vi "UHR-Fleezers Control (host) - 12.1_Jonathan.vi"() -> ()   [LabVIEW 2012] (continued)
        n2038 = xnode "Read/Write Control"("FPGA VI Reference In"=w3388, "error in"=w3383, "FB Reset Set 1"=w3386, "FB Reset Set 2"=w3385) -> ("error out"=w3384:errorcluster)  [unwired: 1 out]
      }
      event "PID Gains": Value Change {
        n2039 = event-data() -> ()  [unwired: 7 out]
        n2040 = Unbundle By Name("PID Gains") -> ("Set 1"=w3392:T15, "Set 2"=w3391:T15)
        n2041 = xnode "Read/Write Control"("FPGA VI Reference In"=w3393, "error in"=w3389, "FB Gains Set 1"=w3392, "FB Gains Set 2"=w3391) -> ("error out"=w3390:errorcluster)  [unwired: 1 out]
      }
      event "AI2 to Setpoint", "Setpoints (V)": Value Change {
        n2042 = event-data() -> ()  [unwired: 7 out]
        n2043 = xnode "Read/Write Control"("FPGA VI Reference In"=w3399, "error in"=w3395) -> ("FPGA VI Reference Out"=w3398:T20, "error out"=w3397:errorcluster, "AI2 Y Sum Set 1"=w3406:i16, "AI2 Y Sum Set 2"=w3405:i16)
        n2044 = Cluster To Array(cluster="AI2 to Setpoint") -> (array=w3409:bool[])
        n2045 = local read "AI2 (V)"() -> (w3407:cluster{"Set 1":dbl, "Set 2":dbl})
        n2046 = Or Array Elements(Boolean array=w3409) -> (logical OR=w3410:bool)
        n2047 = Bundle By Name(cluster=w3407, "Set 1"=w3406, "Set 2"=w3405) -> (w3404:cluster{"Set 1":dbl, "Set 2":dbl})
        n2048 = Divide(x=w3404, y=3276.7) -> (x/y=w3403:cluster{"Set 1":dbl, "Set 2":dbl})
        "AI2 (V)" <- w3403
        n2049 = case shown="True" w3410 {
          tunnel: [w3413 w3430] -> w3402
          tunnel: "AI2 to Setpoint" -> [_ w3426]
          tunnel: "Setpoints (V)" -> [w3414 w3429]
          tunnel: w3403 -> [_ w3423]
          frame False {
            n2050 = Multiply(x=3276.7, y=w3414) -> (x*y=w3415:cluster{"Set 1":dbl, "Set 2":dbl})
            n2051 = To Word Integer(number=w3415) -> (16bit integer=w3413:cluster{"Set 1":i16, "Set 2":i16})
          }
          frame True {
            n2052 = Unbundle By Name(w3423) -> ("Set 1"=w3422:dbl, "Set 2"=w3421:dbl)
            n2053 = Unbundle By Name(w3429) -> ("Set 1"=w3428:dbl, "Set 2"=w3427:dbl)
            n2054 = Unbundle By Name(w3426) -> ("Set 1"=w3425:bool, "Set 2"=w3424:bool)
            n2055 = Select(t=w3422, s=w3425, f=w3428) -> (s? t:f=w3420:dbl)
            n2056 = Select(t=w3421, s=w3424, f=w3427) -> (s? t:f=w3419:dbl)
            n2057 = Bundle By Name(cluster=w3429, "Set 1"=w3420, "Set 2"=w3419) -> (w3417:cluster{"Set 1":dbl, "Set 2":dbl})
            n2058 = local write "Setpoints (V)"(w3417) -> ()
            n2059 = Multiply(x=3276.7, y=w3417) -> (x*y=w3418:cluster{"Set 1":dbl, "Set 2":dbl})
            n2060 = To Word Integer(number=w3418) -> (16bit integer=w3430:cluster{"Set 1":i16, "Set 2":i16})
          }
        }
        n2061 = Unbundle By Name(w3402) -> ("Set 1"=w3401:i16, "Set 2"=w3400:i16)
        n2062 = xnode "Read/Write Control"("FPGA VI Reference In"=w3398, "error in"=w3397, "FB Setpoint Set 1"=w3401, "FB Setpoint Set 2"=w3400) -> ("error out"=w3396:errorcluster)  [unwired: 1 out]
      }
      event "Invert GI": Value Change {
        n2063 = event-data() -> ()  [unwired: 7 out]
        n2064 = xnode "Read/Write Control"("FPGA VI Reference In"=w3435, "error in"=w3433, "Invert GI"="Invert GI", "Invert GI 2"="Invert GI") -> ("error out"=w3434:errorcluster)  [unwired: 1 out]
      }
      event "Green FB Setpoint (mV)", "Green FB Gains", "Green FB On/Off", "Current When FB OFF (%)", "Green int current ON count adj": Value Change {
        n2065 = event-data() -> ()  [unwired: 7 out]
        n2066 = local read "Green FB Setpoint (mV)"() -> (w3442:dbl)
        n2067 = local read "Current When FB OFF (%)"() -> (w3445:dbl)
        n2068 = Multiply(x=w3442, y=3.2767) -> (x*y=w3441:dbl)
        n2069 = Multiply(x=w3445, y=655.35) -> (x*y=w3446:dbl)
        n2070 = To Unsigned Word Integer(number=w3446) -> (unsigned 16bit integer=w3444:u16)
        n2071 = local read "Green int current ON count adj"() -> (w3449:u32)
        n2072 = local read "Green FB Gains"() -> (w3448:T15)
        n2073 = local read "Green Laser ON/Interlacing"() -> (w3439:bool)
        n2074 = local read "Green laser mode"() -> (w3438:enum32{"Laser ON", "Laser OFF", "Interlace"})
        n2075 = local read "Green FB On/Off"() -> (w3450:bool)
        n2076 = Equal?(x=w3438, y=enum32{"Laser ON", "Laser OFF", "Interlace"}."Interlace") -> (x = y?=w3436:bool)
        n2077 = Compound Arithmetic op=AND(w3436, w3450, w3439) -> (w3440:bool)
        n2078 = xnode "Read/Write Control"("FPGA VI Reference In"=w3453, "error in"=w3452, "Green FB Setpoint"=w3441, "Green FB On/Off"=w3440, "Current Out"=w3444, "Green int current ON count adj"=w3449, "Green FB Gains"=w3448) -> ("error out"=w3451:errorcluster)  [unwired: 1 out]
      }
      event "Green laser mode", "Green Laser ON/Interlacing": Value Change {
        n2079 = event-data() -> ()  [unwired: 7 out]
        n2080 = local write "Green Laser ON/OFF"("Green Laser ON/Interlacing") -> ()
        n2081 = case shown="True" "Green Laser ON/Interlacing" {
          tunnel: "Green laser mode" -> [_ w3467]
          tunnel: [enum32{"Laser ON", "Laser OFF", "Interlace"}."Laser OFF" ("Green laser mode") w3467] -> w3456
          tunnel: [FALSE w3463] -> w3455
          frame False {
          }
          frame True {
            n2082 = local read "Green FB On/Off"() -> (w3464:bool)
            n2083 = Equal?(x=w3467, y=enum32{"Laser ON", "Laser OFF", "Interlace"}."Interlace") -> (x = y?=w3465:bool)
            n2084 = And(x=w3465, y=w3464) -> (x .and. y?=w3463:bool)
          }
        }
        n2085 = xnode "Read/Write Control"("FPGA VI Reference In"=w3460, "error in"=w3458, "Operating Mode"=w3456, "Operating Mode 2"=w3456, "Green FB On/Off"=w3455) -> ("error out"=w3459:errorcluster)  [unwired: 1 out]
      }
      event "Green Laser ON/OFF": Value Change {
        n2086 = event-data() -> ()  [unwired: 7 out]
        n2087 = property on="Green Laser ON/Interlacing" class="Bool (strict)"("Val(Sgnl)"="Green Laser ON/OFF") -> ()  [unwired: 2 in, 2 out]
      }
      event "Test ttrig": Value Change {
        n2088 = event-data() -> ()  [unwired: 7 out]
        n2089 = xnode "Read/Write Control"("FPGA VI Reference In"=w3472, "error in"=w3471, "TTrig?"=TRUE) -> ("error out"=w3470:errorcluster)  [unwired: 1 out]
      }
      event "Neg. TTrig FPGA": Value Change {
        n2090 = event-data() -> ()  [unwired: 7 out]
        n2091 = xnode "Read/Write Control"("FPGA VI Reference In"=w3476, "error in"=w3475, "TTrig Negate Pos"="Neg. TTrig FPGA") -> ()  [unwired: 2 out]
      }
      event "- phase (APD 1 Gate)", "+ phase (APD 1 Gate)": Value Change {
        n2092 = event-data() -> ()  [unwired: 7 out]
        n2093 = local read "Phase Adj. (APD 1 Gate)"() -> (w3477:i16)
        n2094 = Negate(x=w3477) -> (-x=w3485:i16)
        n2095 = Select(t=w3485, s="- phase (APD 1 Gate)", f=w3477) -> (s? t:f=w3484:i16)
        n2096 = Or(x="- phase (APD 1 Gate)", y="+ phase (APD 1 Gate)") -> (x .or. y?=w3480:bool)
        n2097 = xnode "Read/Write Control"("FPGA VI Reference In"=w3487, "error in"=w3486, "Phase count adjustment (APD 1 Gate)"=w3484) -> ("FPGA VI Reference Out"=w3482:T20, "error out"=w3483:errorcluster)
        n2098 = xnode "Read/Write Control"("FPGA VI Reference In"=w3482, "error in"=w3483, "+ phase (APD 1 Gate)"=w3480) -> ("error out"=w3481:errorcluster)  [unwired: 1 out]
      }
      event "+ phase (APD 2 Gate)", "- phase (APD 2 Gate)": Value Change {
        n2099 = event-data() -> ()  [unwired: 7 out]
        n2100 = local read "Phase Adj. (APD 2 Gate)"() -> (w3488:i16)
        n2101 = Negate(x=w3488) -> (-x=w3496:i16)
        n2102 = Select(t=w3496, s="- phase (APD 2 Gate)", f=w3488) -> (s? t:f=w3495:i16)
        n2103 = Or(x="- phase (APD 2 Gate)", y="+ phase (APD 2 Gate)") -> (x .or. y?=w3491:bool)
        n2104 = xnode "Read/Write Control"("FPGA VI Reference In"=w3498, "error in"=w3497, "Phase count adjustment (APD 2 Gate)"=w3495) -> ("FPGA VI Reference Out"=w3493:T20, "error out"=w3494:errorcluster)
        n2105 = xnode "Read/Write Control"("FPGA VI Reference In"=w3493, "error in"=w3494, "+ phase (APD 2 Gate)"=w3491) -> ("error out"=w3492:errorcluster)  [unwired: 1 out]
      }
      event "Phase Adj. (APD Acq)", "+ phase (APD Acq)", "- phase (APD Acq)": Value Change {
        n2106 = event-data() -> ()  [unwired: 7 out]
        n2107 = local read "Phase Adj. (APD Acq)"() -> (w3501:i16)
        n2108 = Negate(x=w3501) -> (-x=w3507:i16)
        n2109 = Select(t=w3507, s="+ phase (APD Acq)", f=w3501) -> (s? t:f=w3506:i16)
        n2110 = Or(x="+ phase (APD Acq)", y="- phase (APD Acq)") -> (x .or. y?=w3502:bool)
        n2111 = xnode "Read/Write Control"("FPGA VI Reference In"=w3509, "error in"=w3508, "Phase Count Adjustment (APD Acq)"=w3506) -> ("FPGA VI Reference Out"=w3504:T20, "error out"=w3505:errorcluster)
        n2112 = xnode "Read/Write Control"("FPGA VI Reference In"=w3504, "error in"=w3505, "+ phase (APD Acq)"=w3502) -> ("error out"=w3503:errorcluster)  [unwired: 1 out]
      }
      event "Phase adj. (GI)", "+ phase (GI)", "- phase (GI)": Value Change {
        n2113 = event-data() -> ()  [unwired: 7 out]
        n2114 = Negate(x="Phase adj. (GI)") -> (-x=w3518:i16)
        n2115 = Select(t=w3518, s="+ phase (GI)", f="Phase adj. (GI)") -> (s? t:f=w3517:i16)
        n2116 = Or(x="+ phase (GI)", y="- phase (GI)") -> (x .or. y?=w3513:bool)
        n2117 = xnode "Read/Write Control"("FPGA VI Reference In"=w3520, "error in"=w3519, "Phase count adjustment (GI)"=w3517) -> ("FPGA VI Reference Out"=w3515:T20, "error out"=w3516:errorcluster)
        n2118 = xnode "Read/Write Control"("FPGA VI Reference In"=w3515, "error in"=w3516, "+ phase (GI)"=w3513) -> ("error out"=w3514:errorcluster)  [unwired: 1 out]
      }
      event "Phase adj. (GI) 2", "+ phase (GI) 2", "- phase (GI) 2": Value Change {
        n2119 = event-data() -> ()  [unwired: 7 out]
        n2120 = Negate(x="Phase adj. (GI) 2") -> (-x=w3529:i16)
        n2121 = Select(t=w3529, s="+ phase (GI) 2", f="Phase adj. (GI) 2") -> (s? t:f=w3528:i16)
        n2122 = Or(x="+ phase (GI) 2", y="- phase (GI) 2") -> (x .or. y?=w3524:bool)
        n2123 = xnode "Read/Write Control"("FPGA VI Reference In"=w3531, "error in"=w3530, "Phase count adjustment (GI) 2"=w3528) -> ("FPGA VI Reference Out"=w3526:T20, "error out"=w3527:errorcluster)
        n2124 = xnode "Read/Write Control"("FPGA VI Reference In"=w3526, "error in"=w3527, "+ phase (GI) 2"=w3524) -> ("error out"=w3525:errorcluster)  [unwired: 1 out]
      }
      event "Phase adj. (Green FB)", "- phase (Green FB)", "+ phase (Green FB)": Value Change {
        n2125 = event-data() -> ()  [unwired: 7 out]
        n2126 = Negate(x="Phase adj. (Green FB)") -> (-x=w3540:i16)
        n2127 = Select(t=w3540, s="+ phase (Green FB)", f="Phase adj. (Green FB)") -> (s? t:f=w3539:i16)
        n2128 = Or(x="+ phase (Green FB)", y="- phase (Green FB)") -> (x .or. y?=w3535:bool)
        n2129 = xnode "Read/Write Control"("FPGA VI Reference In"=w3542, "error in"=w3541, "Phase count adjustment (Green FB)"=w3539) -> ("FPGA VI Reference Out"=w3537:T20, "error out"=w3538:errorcluster)
        n2130 = xnode "Read/Write Control"("FPGA VI Reference In"=w3537, "error in"=w3538, "+ phase (Green FB)"=w3535) -> ("error out"=w3536:errorcluster)  [unwired: 1 out]
      }
      event "Invert APD Gate", "APD Gate ON Count", "APD Gate OFF Count", "APD Gate", "APD Integration Time (s)", "APD 1 AO Mult.", "APD 2 AO Mult.", "On one out of X cycles": Value Change {
        n2131 = event-data() -> ()  [unwired: 7 out]
        n2132 = Add(x="GI Frequency, ON count", y="GI Frequency, OFF count") -> (x+y=w3546:u32)
        n2133 = Add(x="APD Gate ON Count", y="APD Gate OFF Count") -> (x+y=w3559:u32)
        n2134 = Multiply(x="On one out of X cycles", y=w3546) -> (x*y=w3543:u32)
        "Green FB Count" <- w3543
        n2135 = Subtract(x=w3543, y="GI Frequency, ON count") -> (x-y=w3544:u32)
        n2136 = Multiply(x=w3559, y="On one out of X cycles") -> (x*y=w3558:u32)
        n2137 = Subtract(x=w3558, y="APD Gate ON Count") -> (x-y=w3557:u32)
        n2138 = local read "DMA Update Period (s)"() -> (w3560:dbl)
        n2139 = Multiply(x="APD Integration Time (s)", y=40000000.0) -> (x*y=w3565:dbl)
        n2140 = Reciprocal(x="APD Integration Time (s)") -> (1/x=→"APD Acq Rate (Hz)":dbl)
        n2141 = To Unsigned Long Integer(number=w3565) -> (unsigned 32bit integer=w3549:u32)
        "APD Int. Count" <- w3549
        n2142 = xnode "Read/Write Control"("FPGA VI Reference In"=w3569, "error in"=w3568, "Invert APD Gate"="Invert APD Gate", "APD Gate ON Count"="APD Gate ON Count", "APD Gate OFF Count"=w3557, "APD Acq Rate Count"=w3549, "APD Gate Operating Mode"="APD Gate", "APD 1 AO scale factor"="APD 1 AO Mult.", "APD 2 AO scale factor"="APD 2 AO Mult.", "Green interlace ON count"="GI Frequency, ON count", "Green interlace OFF count"=w3544, "Green interlace ON count 2"="GI Frequency, ON count", "Green interlace OFF count 2"=w3544, "Green FB Count"=w3543) -> ("error out"=w3567:errorcluster)  [unwired: 1 out]
        n2143 = Divide(x=w3560, y="APD Integration Time (s)") -> (x/y=w3563:dbl)
        n2144 = Multiply(x=2.0, y=w3563) -> (x*y=w3562:dbl)
        n2145 = local write "APD Samples/FIFO Acq."(w3563) -> ()
        n2146 = local write "APD Elements/DMA read"(w3562) -> ()
      }
      event "Number of F/B Scans (AOD)", "Scan Speed (nm/s)", "Scan BD", "Initial delta (MHz)", "Step Size (nm)", "Scan Range (nm)": Value Change {
        w3631 = 123.0  # AOM cal (nm/MHz)
        n2147 = event-data() -> ()  [unwired: 7 out]
        n2148 = local read "BD 1 Frequency 1 (MHz)"() -> (w3614:dbl)
        n2149 = local read "AOM X Cal (nm/MHz)"() -> (w3606:dbl)
        n2150 = local read "X RF Frequency Limits (MHz)"() -> (w3618:T17)
        n2151 = local read "Y RF Frequency Limits (MHz)"() -> (w3615:T17)
        n2152 = local read "BD 2 Frequency 1 (MHz)"() -> (w3620:dbl)
        n2153 = Negate(x="Scan Range (nm)") -> (-x=w3584:dbl)
        n2154 = Divide(x=w3584, y=w3606) -> (x/y=w3588:dbl)
        n2155 = Select(t=w3618, s="Scan BD", f=w3615) -> (s? t:f=w3617:T17)
        n2156 = Select(t=w3614, s="Scan BD", f=w3620) -> (s? t:f=w3619:dbl)
        n2157 = Unbundle By Name(w3617) -> ("Maximum"=w3626:dbl, "Minimum"=w3625:dbl)
        n2158 = Add(x=w3588, y=w3619) -> (x+y=w3623:dbl)
        n2159 = Divide(x=w3584, y="Step Size (nm)") -> (x/y=w3603:dbl)
        n2160 = Divide(x="Step Size (nm)", y=w3606) -> (x/y=w3612:dbl)
        n2161 = Absolute Value(x=w3603) -> (abs(x)=w3587:dbl)
        n2162 = Sign(1:w3584) -> (0:w3585:dbl)
        n2163 = In Range and Coerce(upper limit=w3626, x=w3623, lower limit=w3625) -> (coerced(x)=w3622:dbl, In Range?=w3624:bool)
        n2164 = To Unsigned Quad Integer(1:w3587) -> (0:w3602:u64)
        "Scan steps (AOD)" <- w3602
        n2165 = call "IR AOM freq to word.vi"("Frequency In (MHz)"=w3612) -> ("Frequency Word Out (double)"=w3609:dbl)
        n2166 = Multiply(x=w3585, y=w3609) -> (x*y=w3586:dbl)
        n2167 = Subtract(x=w3623, y=w3622) -> (x-y=w3621:dbl)
        n2168 = To Quad Integer(1:w3586) -> (0:w3608:i64)
        "Incr. int (AOD)" <- w3608
        n2169 = Subtract(x=w3588, y=w3621) -> (x-y=w3607:dbl)
        "Scan Range (MHz)" <- w3607
        n2170 = Select(t=w3588, s=w3624, f=w3607) -> (s? t:f=w3627:dbl)
        n2171 = Multiply(x=w3607, y=w3606) -> (x*y=w3605:dbl)
        n2172 = Decrement(x=w3602) -> (x-1=w3655:u64)
        n2173 = Negate(x=w3605) -> (-x=w3601:dbl)
        n2174 = local write "Scan Range (nm)"(w3601) -> ()
        n2175 = Divide(x=w3627, y=w3655) -> (x/y=w3611:dbl)
        "Scan Increment (MHz)" <- w3611
        n2176 = call "IR AOM freq to word.vi"("Frequency In (MHz)"=w3611) -> ("Frequency Word Out (double)"=w3610:dbl)
        n2177 = Divide(x="Step Size (nm)", y="Scan Speed (nm/s)") -> (x/y=w3598:dbl)
        n2178 = To Quad Integer(1:w3610) -> ()  [unwired: 1 out]
        n2179 = local read "Number Interlace Sets"() -> (w3582:u8)
        n2180 = local read "AI Count (ticks)"() -> (w3583:u32)
        n2181 = local read "Total Counts (ticks)"() -> (w3581:u32)
        n2182 = local read "# Samples/trap"() -> (w3613:u32)
        n2183 = Multiply(x=w3583, y=w3582) -> (x*y=w3580:u32)
        n2184 = Divide(x=w3581, y=w3580) -> (x/y=w3579:dbl)
        n2185 = Select(t=w3614, s="Scan BD", f=w3620) -> (s? t:f=w3652:dbl)
        "Initial freq. (MHz)" <- w3652
        n2186 = Add(x=w3627, y=w3652) -> (x+y=→"Final freq. (MHz)":dbl)
        n2187 = Divide(x=w3581, y=40000000.0) -> (x/y=w3597:dbl)
        n2188 = Divide(x=w3598, y=w3597) -> (x/y=w3596:dbl)
        n2189 = To Unsigned Quad Integer(1:w3596) -> (0:w3571:u64)
        n2190 = Quotient & Remainder(x=w3571, y=u64 2) -> (x-y*floor(x/y)=w3575:u64)  [unwired: 1 out]
        n2191 = Equal?(x=w3575, y=u64 0) -> (x = y?=w3573:bool)
        n2192 = Decrement(x=w3571) -> (x-1=w3572:u64)
        n2193 = Select(t=w3571, s=w3573, f=w3572) -> (s? t:f=w3570:u64)
        "Cycles/step (AOD)" <- w3570
        n2194 = xnode "Read/Write Control"("FPGA VI Reference In"=w3663, "error in"=w3662, "Scan steps"=w3602, "Number of scans"="Number of F/B Scans (AOD)", "Cycles per step"=w3570, "Scan freq.  increment"=w3608, "Scan BD"="Scan BD") -> ("error out"=w3661:errorcluster)  [unwired: 1 out]
        n2195 = Multiply(x=w3602, y=w3570) -> (x*y=w3656:u64)
        n2196 = Multiply(x=w3656, y=u64 2) -> (x*y=w3578:u64)
        n2197 = Multiply(x=w3579, y=w3578) -> (x*y=w3577:dbl)
        "Data points/scan (f/b)" <- w3577
        n2198 = Multiply(x=w3577, y="Number of F/B Scans (AOD)") -> (x*y=w3659:dbl)
        "Data points/scans" <- w3659
        n2199 = Divide(x=w3659, y=w3613) -> (x/y=→"N sets should be saved":dbl)
        n2200 = Multiply(x=w3656, y=w3597) -> (x*y=w3595:dbl)
        "Time/Scan (s) (AOD)" <- w3595
        n2201 = Select(t=w3627, s="Scan BD", f=0.0) -> (s? t:f=w3653:dbl)
        n2202 = Select(t=0.0, s="Scan BD", f=w3627) -> (s? t:f=w3649:dbl)
        n2203 = local read "BD 2 Frequency 2 (MHz)"() -> (w3645:dbl)
        n2204 = local read "BD 1 Frequency 2 (MHz)"() -> (w3648:dbl)
        n2205 = Add(x=w3649, y=w3620) -> (x+y=w3646:dbl)
        n2206 = Add(x=w3614, y=w3653) -> (x+y=w3647:dbl)
        n2207 = Multiply(x=w3595, y=2.0) -> (x*y=w3594:dbl)
        n2208 = Multiply(x=w3594, y="Number of F/B Scans (AOD)") -> (x*y=w3591:dbl)
        n2209 = Divide(x=w3591, y=60.0) -> (x/y=→"Time to Finish All (min)":dbl)
        n2210 = Add(x="Trap 2 Bead Size (nm)", y="Trap 1 Bead Size (nm)") -> (x+y=w3635:dbl)
        n2211 = Divide(x=w3635, y=2.0) -> (x/y=w3629:dbl)
        n2212 = local read "Initial delta (MHz)"() -> (w3632:dbl)
        n2213 = Subtract(x=w3646, y=w3645) -> (x-y=w3643:dbl)
        n2214 = Subtract(x=w3647, y=w3648) -> (x-y=w3644:dbl)
        n2215 = Square(x=w3643) -> (x^2=w3642:dbl)
        n2216 = Square(x=w3644) -> (x^2=w3641:dbl)
        n2217 = Add(x=w3641, y=w3642) -> (x+y=w3640:dbl)
        n2218 = Square Root(x=w3640) -> (sqrt(x)=w3639:dbl)
        "Final delta (MHz)" <- w3639
        n2219 = Multiply(x=w3631, y=w3639) -> (x*y=w3638:dbl)
        n2220 = Multiply(x=w3632, y=w3631) -> (x*y=w3630:dbl)
        n2221 = Subtract(x=w3630, y=w3629) -> (x-y=→"Initial sep (nm)":dbl)
        n2222 = Subtract(x=w3638, y=w3629) -> (x-y=→"Final sep (nm)":dbl)
      }
      event "Freq or Amp switch first", "Swap F1 and F2", "Freq switch delay", "Amp switch delay": Value Change {
        n2223 = event-data() -> ()  [unwired: 7 out]
        n2224 = local read "Freq or Amp switch first"() -> (w3664:bool)
        n2225 = local read "Amp switch delay"() -> (w3665:u16)
        n2226 = local read "Freq switch delay"() -> (w3667:u16)
        n2227 = local read "Swap F1 and F2"() -> (w3666:bool)
        n2228 = xnode "Read/Write Control"("FPGA VI Reference In"=w3670, "error in"=w3669, "Freq switch delay"=w3667, "Swap F1 and F2"=w3666, "Amp switch delay"=w3665, "Freq or Amp switch first"=w3664) -> ("error out"=w3668:errorcluster)  [unwired: 1 out]
      }
      event "Scan steps (MCL)", "Number of scans (MCL)", "Scan Range (V)\n(of steps)", "2D or 1D Scan", "N APD Samp/step", "Fast Scan Dir", "Continuous MCL Scanning", "Scan lines (y)": Value Change {
        w3672 = 32767.0 ("y")
        n2229 = event-data() -> ()  [unwired: 7 out]
        n2230 = Select(t="Scan lines (y)", s="2D or 1D Scan", f="Number of scans (MCL)") -> (s? t:f=w3677:u64)
        n2231 = Decrement(x="Scan steps (MCL)") -> (x-1=w3693:u64)
        n2232 = Divide(x="Scan Range (V)\n(of steps)", y=w3693) -> (x/y=w3692:dbl)
        "Desired Scan Incr (V)" <- w3692
        n2233 = local read "APD Integration Time (s)"() -> (w3685:dbl)
        n2234 = Multiply(x=w3692, y=w3672) -> (x*y=w3701:dbl)
        n2235 = Divide(x=w3701, y=10.0) -> (x/y=w3691:dbl)
        "Desired incr (int)" <- w3691
        n2236 = local read "Update Count (MCL)"() -> (w3697:u32)
        n2237 = Round Toward -Infinity(1:w3691) -> (0:w3700:dbl)
        n2238 = To Word Integer(number=w3700) -> (16bit integer=w3675:i16)
        "Actual Incr. int (MCL)" <- w3675
        n2239 = Multiply(x=w3685, y=40000000.0) -> (x*y=w3698:dbl)
        n2240 = Divide(x=w3698, y=w3697) -> (x/y=w3696:dbl)
        n2241 = Multiply(x=i16 10, y=w3675) -> (x*y=w3673:i16)
        n2242 = Multiply(x="N APD Samp/step", y=w3696) -> (x*y=w3695:dbl)
        "Cycles/step (MCL)" <- w3695
        n2243 = Divide(x=w3673, y=w3672) -> (x/y=→"Actual MCL Inc (V)":dbl)
        n2244 = Multiply(x="N APD Samp/step", y="Scan steps (MCL)") -> (x*y=w3687:dbl)
        n2245 = local read "APD Samples/FIFO Acq."() -> (w3684:dbl)
        n2246 = Multiply(x=w3687, y=u64 2) -> (x*y=w3686:dbl)
        "Data points/scan (f+b)" <- w3686
        n2247 = Multiply(x=w3686, y=w3677) -> (x*y=w3704:dbl)
        "Data points/scans (MCL)" <- w3704
        n2248 = Multiply(x=w3685, y=w3686) -> (x*y=w3678:dbl)
        "Time/f+b scan (s) (MCL)" <- w3678
        n2249 = Divide(x=w3704, y=w3684) -> (x/y=→"N sets should be saved (MCL)":dbl)
        n2250 = Multiply(x=w3678, y=w3677) -> (x*y=→"Total Time (s)":dbl)
        n2251 = Not(x="Fast Scan Dir") -> (.not. x?=w3682:bool)
        n2252 = xnode "Read/Write Control"("FPGA VI Reference In"=w3708, "error in"=w3707, "Scan steps (MCL)"="Scan steps (MCL)", "Number of scans (MCL)"=w3677, "Cycles per step (MCL)"=w3695, "Scan freq.  increment (MCL)"=w3675, "1D or 2D Scan?"="2D or 1D Scan", "MCL Scan Axis"=w3682, "Cont. Scan (MCL)"="Continuous MCL Scanning") -> ("error out"=w3706:errorcluster)  [unwired: 1 out]
      }
      event "Read Cal": Value Change {
        w3710 = 1000.0 ("y")
        n2253 = event-data() -> ()  [unwired: 7 out]
        n2254 = local read "Save file name"() -> (w3735:path)
        n2255 = local write "Read Cal"(FALSE ("Read Cal")) -> ()
        n2256 = Strip Path(path=w3735) -> (stripped path=w3734:path)  [unwired: 1 out]
        n2257 = Path To String(path=w3734) -> (string=w3733:string)
        n2258 = Concatenate Strings(w3733, "\\current.cal" ("string")) -> (w3731:string)
        n2259 = String To Path(string=w3731) -> (path=w3730:path)
        n2260 = Open/Create/Replace File(file path (use dialog)=w3730, operation (0:open)=T37."open", access (0:read/write)=enum16{"read/write", "read-only", "write-only"}."read-only") -> (refnum out=w3738:refnum<file>, error out=w3724:errorcluster)  [unwired: 1 in, 3 out]
        n2261 = Deny Access(4:w3724, 7:w3738) -> (0:w3723:errorcluster, 3:w3729:refnum<file>)  [unwired: 1 out]
        n2262 = Read from Binary File(5:0.0, 8:w3723, 9:T38."big-endian, network order" ("byte order (0:big-endian, network order)"), 10:-1 ("count (1)"), 11:w3729) -> (0:w3722:errorcluster, 2:w3720:dbl[], 3:w3725:refnum<file>)  [unwired: 2 out]
        n2263 = Array To Cluster(array=w3720) -> (cluster=w3719:T49)
        n2264 = Unbundle(w3719) -> ("[0]"=w3718:dbl, "[1]"=w3717:dbl, "[2]"=w3716:dbl, "[3]"=w3715:dbl, "[4]"=w3714:dbl, "[5]"=w3713:dbl)
        n2265 = Close File(refnum=w3725, error in=w3722) -> (error out=→"Read cal error":errorcluster)  [unwired: 1 out]
        n2266 = Multiply(x=w3713, y=w3710) -> (x*y=w3711:dbl)
        n2267 = local write "T2 kappa_x (pN/nm)"(w3715) -> ()
        n2268 = local write "T1 kappa_x (pN/nm)"(w3716) -> ()
        n2269 = local write "T1 alpha_x (nm/V)"(w3718) -> ()
        n2270 = local write "T2 alpha_x (nm/V)"(w3717) -> ()
        n2271 = Multiply(x=w3714, y=w3710) -> (x*y=w3712:dbl)
        n2272 = local write "T1 offset_x (mV)"(w3712) -> ()
        n2273 = local write "T2 offset_x (mV)"(w3711) -> ()
      }
      event "Abort MCL Scan": Value Change {
        n2274 = event-data() -> ()  [unwired: 7 out]
        n2275 = local write "MCL Scanning"(FALSE ("MCL Scanning")) -> ()
        n2276 = xnode "Read/Write Control"("FPGA VI Reference In"=w3743, "error in"=w3742, "Abort scan (MCL)"="Abort MCL Scan") -> ("error out"=w3741:errorcluster)  [unwired: 1 out]
      }
      event "Update Count (MCL)": Value Change {
        n2277 = event-data() -> ()  [unwired: 7 out]
        n2278 = xnode "Read/Write Control"("FPGA VI Reference In"=w3747, "error in"=w3746, "MCL count"="Update Count (MCL)") -> ("error out"=w3745:errorcluster)  [unwired: 1 out]
      }
      event "Phase adjust (MCL)", "+ phase (MCL)", "- phase (MCL)": Value Change {
        n2279 = event-data() -> ()  [unwired: 7 out]
        n2280 = Negate(x="Phase adjust (MCL)") -> (-x=w3756:i16)
        n2281 = Select(t=w3756, s="- phase (MCL)", f="Phase adjust (MCL)") -> (s? t:f=w3754:i16)
        n2282 = Or(x="- phase (MCL)", y="+ phase (MCL)") -> (x .or. y?=w3749:bool)
        n2283 = xnode "Read/Write Control"("FPGA VI Reference In"=w3758, "error in"=w3757, "Phase count adjustment (MCL)"=w3754) -> ("FPGA VI Reference Out"=w3750:T20, "error out"=w3751:errorcluster)
        n2284 = xnode "Read/Write Control"("FPGA VI Reference In"=w3750, "error in"=w3751, "+ phase (MCL)"=w3749) -> ("error out"=w3748:errorcluster)  [unwired: 1 out]
      }
      event "Abort AOD Scan": Value Change {
        n2285 = event-data() -> ()  [unwired: 7 out]
        n2286 = xnode "Read/Write Control"("FPGA VI Reference In"=w3762, "error in"=w3761, "Abort scan"="Abort AOD Scan") -> ("error out"=w3760:errorcluster)  [unwired: 1 out]
      }
      event "Continuous AOD Scanning": Value Change {
        n2287 = event-data() -> ()  [unwired: 7 out]
        n2288 = xnode "Read/Write Control"("FPGA VI Reference In"=w3766, "error in"=w3765, "Cont. Scan"="Continuous AOD Scanning") -> ("error out"=w3764:errorcluster)  [unwired: 1 out]
      }
      event "Index": Value Change {
        n2289 = event-data() -> ()  [unwired: 7 out]
        n2290 = call "Create new save file.vi"("Insert"="", "Ext"=".dat" ("string"), "Index In"="Index") -> ("Path Out"=→"Save file name":path, "Index Out"=w3767:dbl)
        "Save index" <- w3767
        n2291 = local write "Index"(w3767) -> ()
      }
      event "AO1", "AO2": Value Change {
        w3782 = 10.0 ("y")
        w3781 = 32767.0 ("y")
        n2292 = event-data() -> ()  [unwired: 7 out]
        n2293 = local read "AO2"() -> (w3780:dbl)
        n2294 = local read "AO1"() -> (w3777:dbl)
        n2295 = Multiply(x=w3777, y=w3781) -> (x*y=w3776:dbl)
        n2296 = Multiply(x=w3780, y=w3781) -> (x*y=w3779:dbl)
        n2297 = Divide(x=w3776, y=w3782) -> (x/y=w3775:dbl)
        n2298 = Divide(x=w3779, y=w3782) -> (x/y=w3778:dbl)
        n2299 = To Word Integer(number=w3775) -> (16bit integer=w3783:i16)
        n2300 = To Word Integer(number=w3778) -> (16bit integer=w3784:i16)
        n2301 = xnode "Read/Write Control"("FPGA VI Reference In"=w3774, "error in"=w3773, "AO1"=w3783, "AO2"=w3784) -> ("error out"=w3772:errorcluster)  [unwired: 1 out]
      }
      event "Inject Pump 1": Value Change {
        n2302 = event-data() -> ()  [unwired: 7 out]
        n2303 = local read "Use Harvard pumps\nfor beads (else Chemyx)"() -> (w3786:bool)
        n2304 = case shown="True" w3786 {
          tunnel: "Inject Pump 1" -> [w3790 w3828]
          tunnel: w3785 -> [_ w3829]
          frame False {
            n2305 = local read "Pump write delay (ms)"() -> (w3789:dbl)
            n2306 = local read "Chemyx Syringe Pump Serial Port"() -> (w3788:refnum<visa-resource-name>)
            n2307 = case shown="True" w3790 {
              tunnel: w3789 -> [w3796 w3810]
              tunnel: w3788 -> [w3793 w3809]
              frame False {
                n2308 = flat-sequence {
                  tunnel: w3793 -> [w3797]
                  tunnel: [w3797] -> w3794
                  tunnel: w3796 -> [_]
                  tunnel: [w3800] -> w3795
                  tunnel: w3794 -> [w3800]
                  tunnel: w3795 -> [w3801]
                  tunnel: [w3801] -> w3791
                  tunnel: [w3803] -> w3792
                  tunnel: w3791 -> [w3803]
                  tunnel: w3792 -> [w3805]
                  frame #0 {
                    n2309 = call "Write to pump.vi"("string"="enter pump1", "VISA resource name"=w3797) -> ()  [unwired: 1 out]
                  }
                  frame #1 {
                    n2310 = Wait (ms)(milliseconds to wait="Pump pause delay (ms)") -> ()  [unwired: 1 out]
                  }
                  frame #2 {
                    n2311 = call "Write to pump.vi"("string"="stop", "VISA resource name"=w3801) -> ()  [unwired: 1 out]
                  }
                  frame #3 {
                    n2312 = Wait (ms)(milliseconds to wait=u32 500) -> ()  [unwired: 1 out]
                  }
                  frame #4 {
                    n2313 = call "Write to pump.vi"("string"="stop", "VISA resource name"=w3805) -> ()  [unwired: 1 out]
                  }
                }
              }
              frame True {
                n2314 = flat-sequence {
                  tunnel: w3809 -> [w3819]
                  tunnel: w3810 -> [w3814]
                  tunnel: w3810 -> [w3821]
                  tunnel: w3809 -> [w3822]
                  tunnel: [w3822] -> w3807
                  tunnel: [w3824] -> w3808
                  tunnel: w3807 -> [w3824]
                  tunnel: w3808 -> [w3826]
                  frame #0 {
                    n2315 = local read "All Pump Parameters"() -> (w3813:T6)
                    n2316 = Unbundle By Name(w3813) -> ("Pump 1"=w3820:T50)
                    n2317 = call "Set pump parameters.vi"("Pump write delay (ms)"=w3814, "Volume (uL)"="Ch 1 Inject Volume (uL)", "Rate (uL/h)"="Ch 1 Inject Rate (ul/h)", "Units"=4.0, "Pump #"=1.0, "Pump Parameters In"=w3820, "VISA resource name"=w3819) -> ("Pump Parameters Out"=w3812:T50)  [unwired: 3 in]
                    n2318 = Bundle By Name(cluster=w3813, "Pump 1"=w3812) -> (w3811:T6)
                    n2319 = local write "All Pump Parameters"(w3811) -> ()
                  }
                  frame #1 {
                    n2320 = Wait (ms)(milliseconds to wait=w3821) -> ()  [unwired: 1 out]
                  }
                  frame #2 {
                    n2321 = call "Write to pump.vi"("string"="start", "VISA resource name"=w3822) -> ()  [unwired: 1 out]
                  }
                  frame #3 {
                    n2322 = Wait (ms)(milliseconds to wait=u32 500) -> ()  [unwired: 1 out]
                  }
                  frame #4 {
                    n2323 = call "Write to pump.vi"("string"="start", "VISA resource name"=w3826) -> ()  [unwired: 1 out]
                  }
                }
              }
            }
          }
          frame True {
            n2324 = case shown="False" w3828 {
              tunnel: w3829 -> [w3830 w3840]
              frame False {
                n2325 = flat-sequence {
                  tunnel: w3830 -> [w3832]
                  frame #0 {
                    n2326 = local write "Flushing P1"(FALSE ("Flushing P1")) -> ()
                    n2327 = Concatenate Strings("stop" ("string"), "\r") -> (w3834:string)
                    n2328 = VISA Write(VISA resource name=w3832, write buffer=w3834) -> ()  [unwired: 1 in, 3 out]
                  }
                  frame #1 {
                    n2329 = property on="Clear Volume P1" class="Bool (strict)"("Val(Sgnl)"=TRUE ("Value (Signaling)")) -> ()  [unwired: 2 in, 2 out]
                  }
                }
              }
              frame True {
                n2330 = local read "Normal Flow Rate (ul/h) P1"() -> (w3838:dbl)
                n2331 = Number To Decimal String(number=w3838) -> (decimal integer string=w3844:string)  [unwired: 1 in]
                n2332 = Concatenate Strings("irate  " ("string"), w3844, " u/h" ("string"), "\r") -> (w3842:string)
                n2333 = VISA Write(VISA resource name=w3840, write buffer=w3842) -> (VISA resource name out=w3839:refnum<visa-resource-name>)  [unwired: 1 in, 2 out]
                n2334 = Concatenate Strings("irun" ("string"), "\r") -> (w3846:string)
                n2335 = VISA Write(VISA resource name=w3839, write buffer=w3846) -> ()  [unwired: 1 in, 3 out]
              }
            }
          }
        }
      }
      event "Inject Pump 3": Value Change {
        n2336 = event-data() -> ()  [unwired: 7 out]
        n2337 = local read "Use Harvard pumps\nfor beads (else Chemyx)"() -> (w3849:bool)
        n2338 = case shown="True" w3849 {
          tunnel: "Inject Pump 3" -> [w3853 w3892]
          tunnel: w3848 -> [_ w3891]
          frame False {
            n2339 = local read "Pump write delay (ms)"() -> (w3852:dbl)
            n2340 = case shown="True" w3853 {
              tunnel: w3852 -> [w3859 w3873]
              tunnel: "Chemyx Syringe Pump Serial Port" -> [w3856 w3872]
              frame False {
                n2341 = flat-sequence {
                  tunnel: w3856 -> [w3860]
                  tunnel: [w3860] -> w3857
                  tunnel: w3859 -> [_]
                  tunnel: [w3863] -> w3858
                  tunnel: w3857 -> [w3863]
                  tunnel: w3858 -> [w3864]
                  tunnel: [w3864] -> w3854
                  tunnel: [w3866] -> w3855
                  tunnel: w3854 -> [w3866]
                  tunnel: w3855 -> [w3868]
                  frame #0 {
                    n2342 = call "Write to pump.vi"("string"="enter pump3", "VISA resource name"=w3860) -> ()  [unwired: 1 out]
                  }
                  frame #1 {
                    n2343 = local read "Pump pause delay (ms)"() -> (w3862:u32)
                    n2344 = Wait (ms)(milliseconds to wait=w3862) -> ()  [unwired: 1 out]
                  }
                  frame #2 {
                    n2345 = call "Write to pump.vi"("string"="stop", "VISA resource name"=w3864) -> ()  [unwired: 1 out]
                  }
                  frame #3 {
                    n2346 = Wait (ms)(milliseconds to wait=u32 0) -> ()  [unwired: 1 out]
                  }
                  frame #4 {
                    n2347 = call "Write to pump.vi"("string"="stop", "VISA resource name"=w3868) -> ()  [unwired: 1 out]
                  }
                }
              }
              frame True {
                n2348 = flat-sequence {
                  tunnel: w3872 -> [w3882]
                  tunnel: w3873 -> [w3877]
                  tunnel: w3873 -> [w3884]
                  tunnel: w3872 -> [w3885]
                  tunnel: [w3885] -> w3871
                  tunnel: [w3888] -> w3870
                  tunnel: w3871 -> [w3888]
                  tunnel: w3870 -> [w3889]
                  frame #0 {
                    n2349 = local read "All Pump Parameters"() -> (w3876:T6)
                    n2350 = Unbundle By Name(w3876) -> ("Pump 3"=w3883:T50)
                    n2351 = call "Set pump parameters.vi"("Pump write delay (ms)"=w3877, "Volume (uL)"="Ch 3 Inject Volume (uL)", "Rate (uL/h)"="Ch 3 Inject Rate (ul/h)", "Units"=4.0, "Pump #"=3.0, "Pump Parameters In"=w3883, "VISA resource name"=w3882) -> ("Pump Parameters Out"=w3875:T50)  [unwired: 3 in]
                    n2352 = Bundle By Name(cluster=w3876, "Pump 3"=w3875) -> (w3874:T6)
                    n2353 = local write "All Pump Parameters"(w3874) -> ()
                  }
                  frame #1 {
                    n2354 = Wait (ms)(milliseconds to wait=w3884) -> ()  [unwired: 1 out]
                  }
                  frame #2 {
                    n2355 = call "Write to pump.vi"("string"="start", "VISA resource name"=w3885) -> ()  [unwired: 1 out]
                  }
                  frame #3 {
                    n2356 = Wait (ms)(milliseconds to wait=u32 500) -> ()  [unwired: 1 out]
                  }
                  frame #4 {
                    n2357 = call "Write to pump.vi"("string"="start", "VISA resource name"=w3889) -> ()  [unwired: 1 out]
                  }
                }
              }
            }
          }
          frame True {
            n2358 = case shown="False" w3892 {
              tunnel: w3891 -> [w3893 w3900]
              frame False {
                n2359 = flat-sequence {
                  tunnel: w3893 -> [w3895]
                  frame #0 {
                    n2360 = local write "Flushing P3"(FALSE ("Flushing P3")) -> ()
                    n2361 = Concatenate Strings("stop" ("string"), "\r") -> (w3897:string)
                    n2362 = VISA Write(VISA resource name=w3895, write buffer=w3897) -> ()  [unwired: 1 in, 3 out]
                  }
                  frame #1 {
                    n2363 = property on="Clear Volume P3" class="Bool (strict)"("Val(Sgnl)"=TRUE ("Value (Signaling)")) -> ()  [unwired: 2 in, 2 out]
                  }
                }
              }
              frame True {
                n2364 = local read "Normal Flow Rate (ul/h) P3"() -> (w3901:dbl)
                n2365 = Number To Decimal String(number=w3901) -> (decimal integer string=w3907:string)  [unwired: 1 in]
                n2366 = Concatenate Strings("irate  " ("string"), w3907, " u/h" ("string"), "\r") -> (w3905:string)
                n2367 = VISA Write(VISA resource name=w3900, write buffer=w3905) -> (VISA resource name out=w3903:refnum<visa-resource-name>)  [unwired: 1 in, 2 out]
                n2368 = Concatenate Strings("irun" ("string"), "\r") -> (w3909:string)
                n2369 = VISA Write(VISA resource name=w3903, write buffer=w3909) -> ()  [unwired: 1 in, 3 out]
              }
            }
          }
        }
      }
      event "Inject Pump 2": Value Change {
        n2370 = event-data() -> ()  [unwired: 7 out]
        n2371 = local read "Pump write delay (ms)"() -> (w3913:dbl)
        n2372 = flat-sequence {
          tunnel: w3911 -> [w3926]
          tunnel: w3913 -> [w3922]
          tunnel: "Inject Pump 2" -> [_]
          tunnel: w3913 -> [w3928]
          tunnel: w3911 -> [w3929]
          frame #0 {
            n2373 = local read "All Pump Parameters"() -> (w3921:T6)
            n2374 = Multiply(x=60.0, y="Flush Center Ch Rate (ul/m)") -> (x*y=w3918:dbl)
            n2375 = Unbundle By Name(w3921) -> ("Pump 2"=w3927:T50)
            n2376 = call "Set pump parameters.vi"("Pump write delay (ms)"=w3922, "Volume (uL)"="Flush Center Ch Volume (uL)", "Rate (uL/h)"=w3918, "Units"=3.0, "Pump #"=2.0, "Pump Parameters In"=w3927, "VISA resource name"=w3926) -> ("Pump Parameters Out"=w3920:T50)  [unwired: 3 in]
            n2377 = Bundle By Name(cluster=w3921, "Pump 2"=w3920) -> (w3919:T6)
            n2378 = local write "All Pump Parameters"(w3919) -> ()
            n2379 = Add(x="Flush Center Ch Volume (uL)", y="Total Volume\nFlushed (uL)") -> (x+y=w3915:dbl)
            n2380 = local write "Total Volume\nFlushed (uL)"(w3915) -> ()
          }
          frame #1 {
            n2381 = Wait (ms)(milliseconds to wait=w3928) -> ()  [unwired: 1 out]
          }
          frame #2 {
            n2382 = call "Write to pump.vi"("string"="start", "VISA resource name"=w3929) -> ()  [unwired: 1 out]
          }
        }
        n2383 = local read "Chemyx Syringe Pump Serial Port"() -> (w3911:refnum<visa-resource-name>)
      }
      event "Sample Channel\nFlow": Value Change {
        n2384 = event-data() -> ()  [unwired: 7 out]
        n2385 = Select(t="irun" ("string"), s="Sample Channel\nFlow", f="stop" ("string")) -> (s? t:f=w3933:string)
        n2386 = Concatenate Strings(w3933, "\r") -> (w3936:string)
        n2387 = VISA Write(VISA resource name=w3931, write buffer=w3936) -> ()  [unwired: 1 in, 3 out]
      }
      event "Start Flow": Value Change {
        n2388 = event-data() -> ()  [unwired: 7 out]
        n2389 = local write "Sample Channel\nFlow"(TRUE ("Sample Channel\nFlow")) -> ()
        n2390 = local write "Start Flow"(FALSE ("Start Flow")) -> ()
        n2391 = Concatenate Strings("irun" ("string"), "\r") -> (w3942:string)
        n2392 = VISA Write(VISA resource name=w3938, write buffer=w3942) -> ()  [unwired: 1 in, 3 out]
      }
      event "Stop Flow": Value Change {
        w3944 = FALSE ("Stop Flow")
        n2393 = event-data() -> ()  [unwired: 7 out]
        n2394 = local write "Stop Flow"(w3944) -> ()
        n2395 = local write "Sample Channel\nFlow"(w3944) -> ()
        n2396 = Concatenate Strings("stop" ("string"), "\r") -> (w3947:string)
        n2397 = VISA Write(VISA resource name=w3945, write buffer=w3947) -> ()  [unwired: 1 in, 3 out]
      }
      event "Flow rate (uL/h)": Value Change {
        n2398 = event-data() -> ()  [unwired: 7 out]
        n2399 = Number To Decimal String(number="Flow rate (uL/h)") -> (decimal integer string=w3954:string)  [unwired: 1 in]
        n2400 = Concatenate Strings("irate  " ("string"), w3954, " u/h" ("string"), "\r") -> (w3953:string)
        n2401 = VISA Write(VISA resource name=w3950, write buffer=w3953) -> ()  [unwired: 1 in, 3 out]
      }
      event "Flush Sample": Value Change {
        n2402 = event-data() -> ()  [unwired: 7 out]
        n2403 = flat-sequence {
          tunnel: w3959 -> [w3987]
          tunnel: [w3967] -> w3958
          tunnel: [w3961] -> w3956
          tunnel: w3958 -> [w3991]
          tunnel: [w3991] -> w3957
          tunnel: w3956 -> [w3990]
          tunnel: w3957 -> [w3996]
          frame #0 {
            # "set paramaters (rate, volume) for flush, clear volume"
            n2404 = Number To Decimal String(number="Flush rate (uL/m)") -> (decimal integer string=w3983:string)  [unwired: 1 in]
            n2405 = Concatenate Strings("irate  " ("string"), w3983, " u/m" ("string"), "\r") -> (w3985:string)
            n2406 = VISA Write(VISA resource name=w3987, write buffer=w3985) -> (VISA resource name out=w3981:refnum<visa-resource-name>)  [unwired: 1 in, 2 out]
            n2407 = Reciprocal(x="Flush rate (uL/m)") -> (1/x=w3964:dbl)
            n2408 = Number To Decimal String(number="Volume (uL)") -> (decimal integer string=w3972:string)  [unwired: 1 in]
            n2409 = Multiply(x="Volume (uL)", y=w3964) -> (x*y=w3963:dbl)
            n2410 = Concatenate Strings("tvolume  " ("string"), w3972, " u" ("string"), "\r") -> (w3970:string)
            n2411 = Multiply(x=w3963, y=60000.0) -> (x*y=w3961:dbl)
            n2412 = VISA Write(VISA resource name=w3981, write buffer=w3970) -> (VISA resource name out=w3969:refnum<visa-resource-name>)  [unwired: 1 in, 2 out]
            n2413 = Concatenate Strings("cvolume" ("string"), "\r") -> (w3968:string)
            n2414 = VISA Write(VISA resource name=w3969, write buffer=w3968) -> (VISA resource name out=w3979:refnum<visa-resource-name>)  [unwired: 1 in, 2 out]
            n2415 = Concatenate Strings("irun" ("string"), "\r") -> (w3977:string)
            n2416 = VISA Write(VISA resource name=w3979, write buffer=w3977) -> (VISA resource name out=w3967:refnum<visa-resource-name>)  [unwired: 1 in, 2 out]
          }
          frame #1 {
            # "Have to wait until\nflow is done to reset\nrate"
            n2417 = Add(x=w3990, y=100.0) -> (x+y=w3989:dbl)
            n2418 = Wait (ms)(milliseconds to wait=w3989) -> ()  [unwired: 1 out]
          }
          frame #2 {
            # "reset flow rate to usual flow rate"
            n2419 = local read "Flow rate (uL/h)"() -> (w4002:dbl)
            n2420 = Number To Decimal String(number=w4002) -> (decimal integer string=w4000:string)  [unwired: 1 in]
            n2421 = Concatenate Strings("irate  " ("string"), w4000, " u/h" ("string"), "\r") -> (w3998:string)
            n2422 = VISA Write(VISA resource name=w3996, write buffer=w3998) -> (VISA resource name out=w3992:refnum<visa-resource-name>)  [unwired: 1 in, 2 out]
            n2423 = Concatenate Strings("cvolume" ("string"), "\r") -> (w3993:string)
            n2424 = VISA Write(VISA resource name=w3992, write buffer=w3993) -> ()  [unwired: 1 in, 3 out]
          }
        }
      }
      event "Flush Pump 3": Value Change {
        n2425 = event-data() -> ()  [unwired: 7 out]
        n2426 = flat-sequence {
          tunnel: w4003 -> [w4006]
          frame #0 {
            # "set paramaters (rate, volume) for flush, clear volume"
            n2427 = Number To Decimal String(number="Flush rate (uL/m) P3") -> (decimal integer string=w4028:string)  [unwired: 1 in]
            n2428 = local write "Inject Pump 3"(TRUE ("Inject Pump 3")) -> ()
            n2429 = Concatenate Strings("irate  " ("string"), w4028, " u/m" ("string"), "\r") -> (w4030:string)
            n2430 = VISA Write(VISA resource name=w4006, write buffer=w4030) -> (VISA resource name out=w4026:refnum<visa-resource-name>)  [unwired: 1 in, 2 out]
            n2431 = Reciprocal(x="Flush rate (uL/m) P3") -> (1/x=w4010:dbl)
            n2432 = Number To Decimal String(number="Volume (uL) P3") -> (decimal integer string=w4017:string)  [unwired: 1 in]
            n2433 = Multiply(x="Volume (uL) P3", y=w4010) -> (x*y=w4009:dbl)
            n2434 = Concatenate Strings("tvolume  " ("string"), w4017, " u" ("string"), "\r") -> (w4015:string)
            n2435 = Multiply(x=w4009, y=60.0) -> (x*y=→"HP3 Flush Time (s)":dbl)
            n2436 = VISA Write(VISA resource name=w4026, write buffer=w4015) -> (VISA resource name out=w4014:refnum<visa-resource-name>)  [unwired: 1 in, 2 out]
            n2437 = Concatenate Strings("cvolume" ("string"), "\r") -> (w4013:string)
            n2438 = VISA Write(VISA resource name=w4014, write buffer=w4013) -> (VISA resource name out=w4024:refnum<visa-resource-name>)  [unwired: 1 in, 2 out]
            n2439 = Concatenate Strings("irun" ("string"), "\r") -> (w4022:string)
            n2440 = VISA Write(VISA resource name=w4024, write buffer=w4022) -> ()  [unwired: 1 in, 3 out]
          }
          frame #1 {
            "Flushing P3" <- TRUE ("Flushing P3")
          }
        }
      }
      event "Flush Pump 1": Value Change {
        n2441 = event-data() -> ()  [unwired: 7 out]
        n2442 = flat-sequence {
          tunnel: [w4044] -> w4034
          tunnel: w4033 -> [w4037]
          tunnel: w4034 -> [_]
          frame #0 {
            # "set paramaters (rate, volume) for flush, clear volume"
            n2443 = local write "Inject Pump 1"(TRUE ("Inject Pump 1")) -> ()
            n2444 = Number To Decimal String(number="Flush rate (uL/m) P1") -> (decimal integer string=w4060:string)  [unwired: 1 in]
            n2445 = Concatenate Strings("irate  " ("string"), w4060, " u/m" ("string"), "\r") -> (w4062:string)
            n2446 = VISA Write(VISA resource name=w4037, write buffer=w4062) -> (VISA resource name out=w4058:refnum<visa-resource-name>)  [unwired: 1 in, 2 out]
            n2447 = Reciprocal(x="Flush rate (uL/m) P1") -> (1/x=w4041:dbl)
            n2448 = Number To Decimal String(number="Volume (uL) P1") -> (decimal integer string=w4049:string)  [unwired: 1 in]
            n2449 = Multiply(x="Volume (uL) P1", y=w4041) -> (x*y=w4040:dbl)
            n2450 = Concatenate Strings("tvolume  " ("string"), w4049, " u" ("string"), "\r") -> (w4047:string)
            n2451 = Multiply(x=w4040, y=60.0) -> (x*y=→"HP1 Flush Time (s)":dbl)
            n2452 = VISA Write(VISA resource name=w4058, write buffer=w4047) -> (VISA resource name out=w4046:refnum<visa-resource-name>)  [unwired: 1 in, 2 out]
            n2453 = Concatenate Strings("cvolume" ("string"), "\r") -> (w4045:string)
            n2454 = VISA Write(VISA resource name=w4046, write buffer=w4045) -> (VISA resource name out=w4056:refnum<visa-resource-name>)  [unwired: 1 in, 2 out]
            n2455 = Concatenate Strings("irun" ("string"), "\r") -> (w4054:string)
            n2456 = VISA Write(VISA resource name=w4056, write buffer=w4054) -> (VISA resource name out=w4044:refnum<visa-resource-name>)  [unwired: 1 in, 2 out]
          }
          frame #1 {
            "Flushing P1" <- TRUE ("Flushing P3")
          }
        }
      }
      event "Clear Volume": Value Change {
        n2457 = event-data() -> ()  [unwired: 7 out]
        n2458 = Concatenate Strings("cvolume" ("string"), "\r") -> (w4066:string)
        n2459 = VISA Write(VISA resource name=w4065, write buffer=w4066) -> ()  [unwired: 1 in, 3 out]
      }
      event "Clear Volume P3": Value Change {
        n2460 = event-data() -> ()  [unwired: 7 out]
        n2461 = Concatenate Strings("cvolume" ("string"), "\r") -> (w4072:string)
        n2462 = VISA Write(VISA resource name=w4071, write buffer=w4072) -> ()  [unwired: 1 in, 3 out]
        n2463 = local write "Clear Volume P3"(FALSE ("Clear Volume P3")) -> ()
      }
      event "Clear Volume P1": Value Change {
        n2464 = event-data() -> ()  [unwired: 7 out]
        n2465 = Concatenate Strings("cvolume" ("string"), "\r") -> (w4077:string)
        n2466 = local write "Clear Volume P1"(FALSE ("Clear Volume P1")) -> ()
        n2467 = VISA Write(VISA resource name=w4076, write buffer=w4077) -> ()  [unwired: 1 in, 3 out]
      }
      event "Display On P3": Value Change {
        n2468 = event-data() -> ()  [unwired: 7 out]
        n2469 = Select(t="dim 100", s="Display On P3", f="dim 0") -> (s? t:f=w4083:string)
        n2470 = Concatenate Strings(w4083, "\r") -> (w4085:string)
        n2471 = VISA Write(VISA resource name=w4080, write buffer=w4085) -> ()  [unwired: 1 in, 3 out]
      }
      event "Display On P1": Value Change {
        n2472 = event-data() -> ()  [unwired: 7 out]
        n2473 = Select(t="dim 100", s="Display On P1", f="dim 0") -> (s? t:f=w4090:string)
        n2474 = Concatenate Strings(w4090, "\r") -> (w4092:string)
        n2475 = VISA Write(VISA resource name=w4087, write buffer=w4092) -> ()  [unwired: 1 in, 3 out]
      }
      event "Retract Pump 3": Value Change {
        n2476 = event-data() -> ()  [unwired: 7 out]
        n2477 = local write "Retract Pump 3"(FALSE ("Retract Pump 3")) -> ()
        n2478 = case shown="True" "Retract Pump 3" {
          tunnel: w4094 -> [_ w4097]
          frame False {
          }
          frame True {
            n2479 = Number To Decimal String(number="Retract Rate (uL/m)") -> (decimal integer string=w4115:string)  [unwired: 1 in]
            n2480 = Concatenate Strings("wrate  " ("string"), w4115, " u/m" ("string"), "\r") -> (w4117:string)
            n2481 = VISA Write(VISA resource name=w4097, write buffer=w4117) -> (VISA resource name out=w4108:refnum<visa-resource-name>)  [unwired: 1 in, 2 out]
            n2482 = Number To Decimal String(number="Retract Vol 3 (uL)") -> (decimal integer string=w4110:string)  [unwired: 1 in]
            n2483 = Concatenate Strings("tvolume  " ("string"), w4110, " u" ("string"), "\r") -> (w4107:string)
            n2484 = VISA Write(VISA resource name=w4108, write buffer=w4107) -> (VISA resource name out=w4103:refnum<visa-resource-name>)  [unwired: 1 in, 2 out]
            n2485 = Concatenate Strings("cvolume" ("string"), "\r") -> (w4104:string)
            n2486 = VISA Write(VISA resource name=w4103, write buffer=w4104) -> (VISA resource name out=w4098:refnum<visa-resource-name>)  [unwired: 1 in, 2 out]
            n2487 = Concatenate Strings("wrun" ("string"), "\r") -> (w4099:string)
            n2488 = VISA Write(VISA resource name=w4098, write buffer=w4099) -> ()  [unwired: 1 in, 3 out]
          }
        }
      }
      event "Retract Pump 1": Value Change {
        n2489 = event-data() -> ()  [unwired: 7 out]
        n2490 = local write "Retract Pump 1"(FALSE ("Retract Pump 1")) -> ()
        n2491 = case shown="True" "Retract Pump 1" {
          tunnel: w4119 -> [_ w4124]
          frame False {
          }
          frame True {
            n2492 = local read "Retract Rate (uL/m)"() -> (w4122:dbl)
            n2493 = Number To Decimal String(number=w4122) -> (decimal integer string=w4140:string)  [unwired: 1 in]
            n2494 = Concatenate Strings("wrate  " ("string"), w4140, " u/m" ("string"), "\r") -> (w4142:string)
            n2495 = VISA Write(VISA resource name=w4124, write buffer=w4142) -> (VISA resource name out=w4134:refnum<visa-resource-name>)  [unwired: 1 in, 2 out]
            n2496 = Number To Decimal String(number="Retract Vol 1 (uL)") -> (decimal integer string=w4136:string)  [unwired: 1 in]
            n2497 = Concatenate Strings("tvolume  " ("string"), w4136, " u" ("string"), "\r") -> (w4133:string)
